vi "Store Data.vi"(6 "All Data":dbl[][](array[numeric]), 7 "Block Size":i32=10, 8 "error in":errorcluster, 9 "File Name":string, 10 "Byte Stream File in":refnum<file>, 11 "Instrument List In":T1[](array[typedef]) {"Private"."Offset" format="%^_3e"; "Private"."Scale Factors" format="%^_3e"}) -> (0 "error out":errorcluster, 3 "Instrument List Out":T1[](array[typedef]) {"Private"."Offset" format="%^_3e"; "Private"."Scale Factors" format="%^_3e"})   [LabVIEW 2021]
uses:
  Sub Controls/Instrument Properties.ctl
  Sub Controls/Public.ctl
  Sub Controls/Private.ctl
  Sub Controls/Instrument Ref.ctl
  Sub Controls/SystemCheckBox-resize.ctl
panel:
  # "Row"
  # "Col"
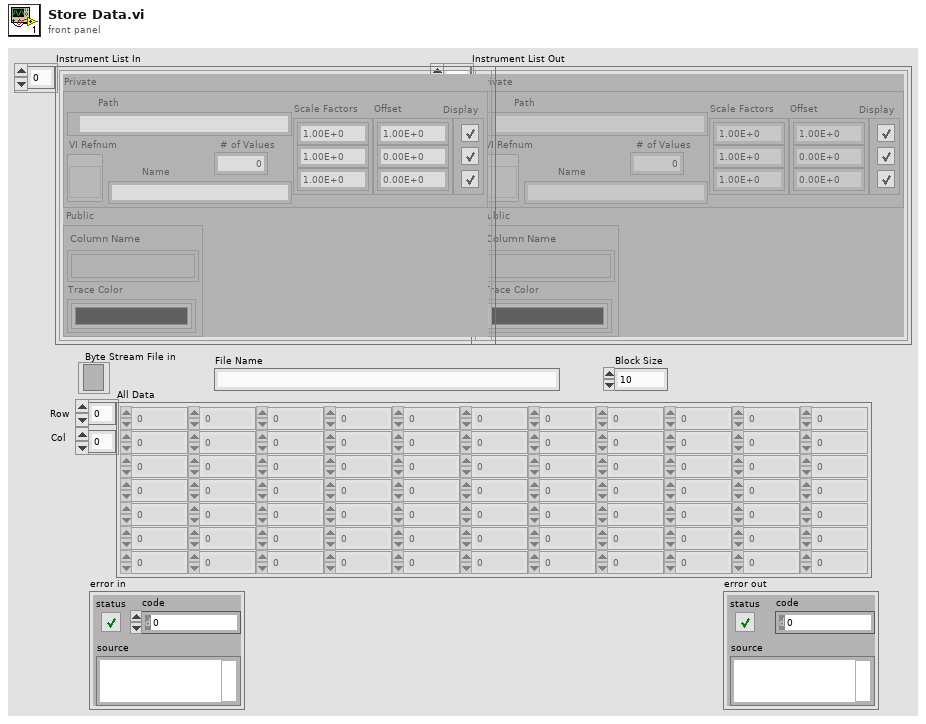
[diagram p1: front panel]
types:
  T1 = typedef "Instrument Properties.ctl" = cluster{"Public":T2, "Private":T3}
  T2 = typedef "Public.ctl" = cluster{"Column Name":string[], "Trace Color":u32[]}
  T3 = typedef "Private.ctl" = cluster{"Path":path, "VI Refnum":T4, "Name":string, "# of Values":i32, "Scale Factors":dbl[], "Display":T5[], "Offset":dbl[]}
  T4 = typedef "Instrument Ref.ctl" = refnum<vi>
  T5 = typedef "SystemCheckBox-resize.ctl" = bool
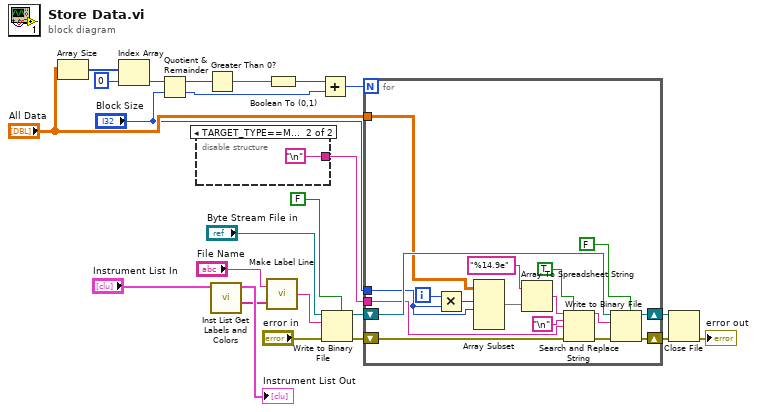
[diagram p0: block diagram]
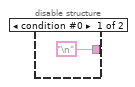
[diagram p2: hidden frame]
diagram:
  n1 = Array Size(array="All Data") -> (size(s)=w12:i32[])
  n2 = Index Array(array=w12, index=0) -> (element=w9:i32)
  n3 = Quotient & Remainder(x=w9, y="Block Size") -> (x-y*floor(x/y)=w5:i32, floor(x/y)=w10:i32)
  n4 = disable-structure shown="TARGET_TYPE==Mac" {
    disable-tunnel: ["\n" "\n"] -> w22
    frame condition #0 {
    }
    frame condition #1 (active) {
    }
  }
  n5 = Greater Than 0?(x=w5) -> (x > 0?=w8:bool)
  n6 = call "Inst List Get Labels and Colors.vi"("Instrument List"="Instrument List In") -> ("Labels"=w14:string[], "Instrument List Out"=→"Instrument List Out":T1[])  [unwired: 4 in, 5 out]
  n7 = call "Make Label Line.vi"("Column Names"=w14, "File Name"="File Name") -> ("Igor Column Headings"=w19:string)
  n8 = Boolean To (0,1)(Boolean=w8) -> (0, 1=w6:i16)
  n9 = Add(x=w6, y=w10) -> (x+y=w7:i32)
  n10 = Write to Binary File(file (use dialog)="Byte Stream File in", data=w19, error in="error in", 5:FALSE ("prepend array or string size? (T)")) -> (refnum out=w16:refnum<file>, error out=w3:errorcluster)  [unwired: 2 in, 1 out]
  n11 = for {
    N: w7 -> [_]
    tunnel: "All Data" -> [w35]
    tunnel: w22 -> [w36]
    tunnel: "Block Size" -> [w31]
    shift-right: [w42] -> w17
    shift-left: w16 -> [w41]
    shift-right: [w28] -> w2
    shift-left: w3 -> [w30]
    i -> [w33]
    n12 = Multiply(x=w33, y=w31) -> (x*y=w32:i32)
    n13 = Array Subset(array=w35, index (row)=w32, length (row)=w31) -> (w34:dbl[][])  [unwired: 2 in]
    n14 = Array To Spreadsheet String(array=w34, 3:"%14.9e") -> (spreadsheet string=w38:string)  [unwired: 1 in]
    n15 = Search and Replace String(replace all?=TRUE ("replace all? (F)"), input string=w38, search string="\n", replace string=w36, error in=w30) -> (result string=w39:string, error out=w29:errorcluster)  [unwired: 3 in, 2 out]
    n16 = Write to Binary File(file (use dialog)=w41, data=w39, error in=w29, 5:FALSE ("prepend array or string size? (T)")) -> (refnum out=w42:refnum<file>, error out=w28:errorcluster)  [unwired: 2 in, 1 out]
  }
  n17 = Close File(refnum=w17, error in=w2) -> (error out=→"error out":errorcluster)  [unwired: 1 out]
